vi "Create test signal for THD.vi"(5 "block size":i32=512, 6 "1mV at 60 Hz":bool, 7 "sampling frequency (Hz)":dbl=51200.0, 9 "noise level (Vrms)":dbl(slide) scale=0.0..10.0, 10 "fundamental amplitude":dbl=1.0, 11 "fundamental frequency (Hz)":dbl=1234.0) -> (3 "Test signal":waveform(dbl)(graph))   [LabVIEW 2020]
doc: "Create a test signal using a polynomial to simulate nonlinear distortion."
uses:
  <vilib>/Analysis/NI_AALBase.lvlib
panel:
  in  "DC level":dbl
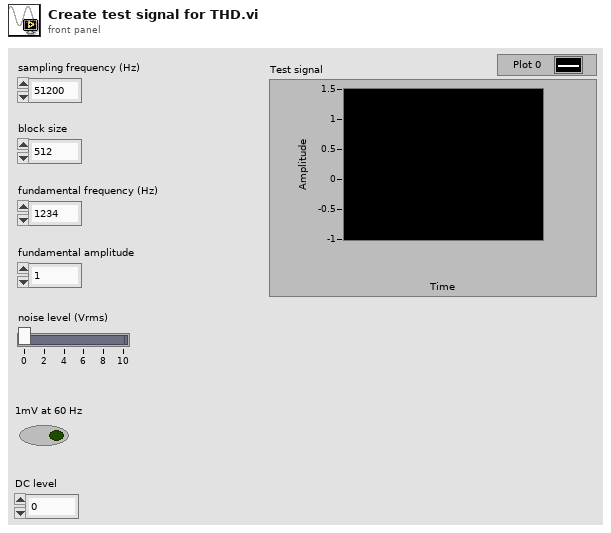
[diagram p1: front panel]
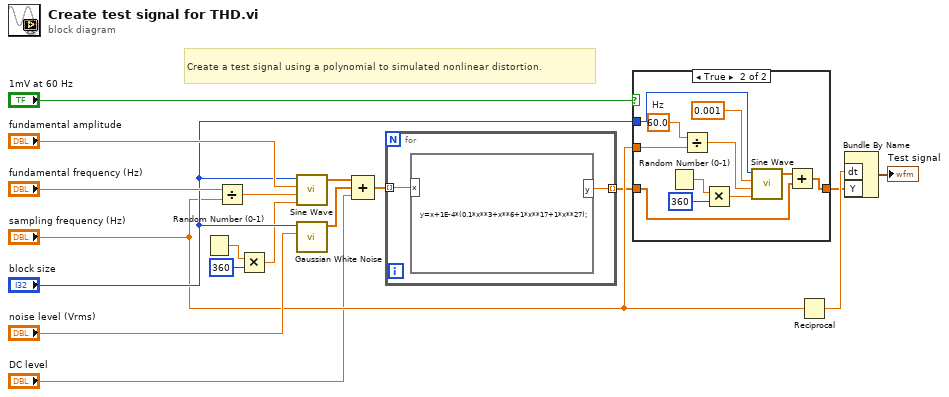
[diagram p0: block diagram]
diagram:
  # "Create a test signal using a polynomial to simulated nonlinear distortion."
  n1 = Random Number (0-1)() -> (number: 0 to 1=w17:dbl)
  n2 = Divide(x="fundamental frequency (Hz)", y="sampling frequency (Hz)") -> (x/y=w4:dbl)
  n3 = Multiply(x=w17, y=360) -> (x*y=w5:dbl)
  n4 = call <vilib>:"Sine Wave.vi"("samples"="block size", "amplitude"="fundamental amplitude", "frequency"=w4, "phase in"=w5) -> ("sine wave"=w11:dbl[])  [unwired: 1 in, 2 out]
  n5 = call <vilib>:"Gaussian White Noise.vi"("standard deviation"="noise level (Vrms)", "samples"="block size") -> ("Gaussian noise pattern"=w3:dbl[])  [unwired: 8 in, 1 out]
  n6 = Compound Arithmetic op=ADD(w11, w3, "DC level") -> (w9:dbl[])
  n7 = for {
    tunnel: w9 -> [w20] mode=indexing
    tunnel: [w19] -> w10 mode=indexing
    n8 = formula code="y=x+1E-4*(0.1*x**3+x**6+1*x**17+1*x**27);"("x"=w20) -> ("y"=w19:dbl)
  }
  n9 = case shown="True" "1mV at 60 Hz" {
    tunnel: "block size" -> [_ w27]
    tunnel: "sampling frequency (Hz)" -> [_ w28]
    tunnel: w10 -> [w21 w31]
    tunnel: [w21 w29] -> w7
    frame False {
    }
    frame True {
      w24 = 60.0  # Hz
      n10 = Random Number (0-1)() -> (number: 0 to 1=w32:dbl)
      n11 = Divide(x=w24, y=w28) -> (x/y=w25:dbl)
      n12 = Multiply(x=w32, y=360) -> (x*y=w26:dbl)
      n13 = call <vilib>:"Sine Wave.vi"("samples"=w27, "amplitude"=0.001, "frequency"=w25, "phase in"=w26) -> ("sine wave"=w30:dbl[])  [unwired: 1 in, 2 out]
      n14 = Add(x=w30, y=w31) -> (x+y=w29:dbl[])
    }
  }
  n15 = Reciprocal(x="sampling frequency (Hz)") -> (1/x=w8:dbl)
  n16 = Bundle By Name("dt"=w8, "Y"=w7) -> (→"Test signal":waveform(dbl))  [unwired: 1 in]
